vi "Open if Invalid Reference.vi"(8 "error in (no error)":errorcluster, 10 "refnum":T1, 11 "Process in":refnum<class "Process.lvclass">) -> (0 "error out":errorcluster, 1 "File opened?":bool, 2 "refnum out":T1, 3 "Process out":refnum<class "Process.lvclass">)   [LabVIEW 2020, in "Configuration File.lvlib"]
uses:
  Configuration File.lvlib
  <vilib>/Utility/config.llb/NI_LVConfig.lvlib
  Process Classes/Process/Process.lvclass
  <vilib>/Utility/config.llb/Config Data RefNum.ctl
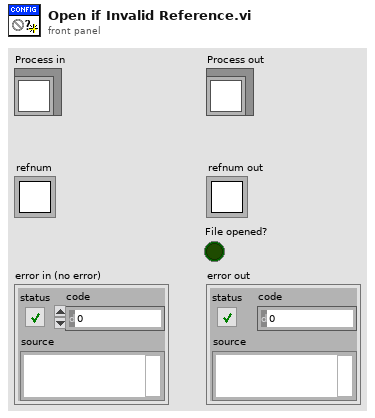
[diagram p1: front panel]
types:
  T1 = typedef "NI_LVConfig.lvlib/Config Data RefNum.ctl" = refnum<k1>
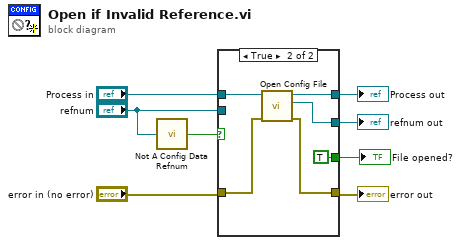
[diagram p0: block diagram]
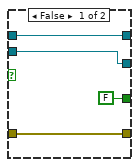
[diagram p2: hidden frame]
diagram:
  n1 = call <vilib>:"Not A Config Data Refnum.vi"("refnum"="refnum") -> ("not a config data refnum"=w5:bool)
  n2 = case shown="True" w5 {
    tunnel: [w12 w18] -> w2
    tunnel: "error in (no error)" -> [w11 w17]
    tunnel: [w11 w16] -> w4
    tunnel: "refnum" -> [w12 _]
    tunnel: [w10 w15] -> w7
    tunnel: "Process in" -> [w10 w14]
    tunnel: [FALSE TRUE] -> w1
    frame False {
    }
    frame True {
      n3 = call "Open Config File.vi"("error in (no error)"=w17, "Process in"=w14) -> ("error out"=w16:errorcluster, "refnum out"=w18:T1, "Process out"=w15:refnum<class "Process.lvclass">)  [unwired: 6 in, 1 out]
    }
  }
  "Process out" <- w7
  "error out" <- w4
  "refnum out" <- w2
  "File opened?" <- w1
